vi "Get Control Terminals.vi"(8 "error in (no error)":errorcluster, 11 "VI in":refnum<vi>) -> (0 "error out":errorcluster, 2 "Controls":map{string, refnum<vi>}(c390), 3 "VI out":refnum<vi>)   [LabVIEW 2020, in "Pure Mock Class Generator.lvclass"]
uses:
  Pure Mock Class Generator.lvclass
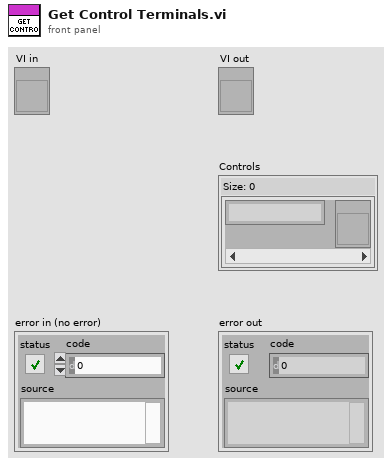
[diagram p1: front panel]
types:
  T1 = enum16{"Invalid Wire Rule", "Required", "Recommended", "Optional", "Dynamic Dispatch"}[]
  T2 = enum16{"Invalid Wire Rule", "Required", "Recommended", "Optional", "Dynamic Dispatch"}
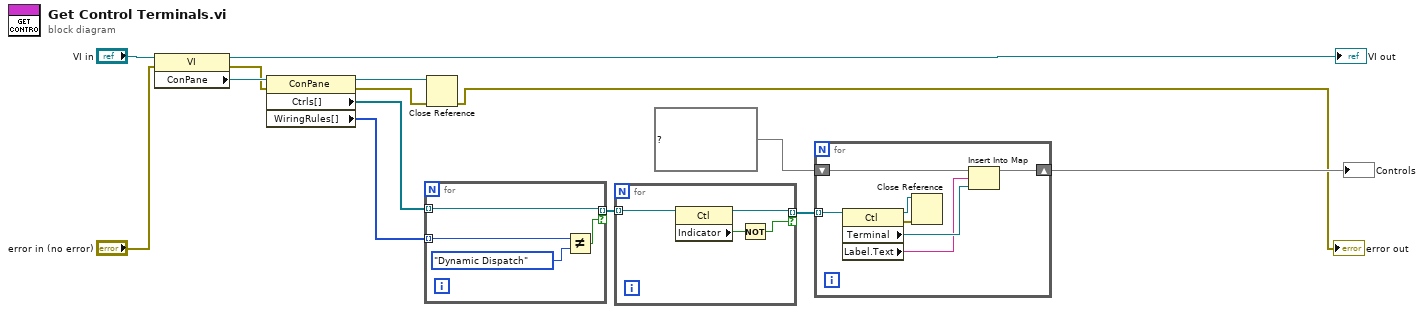
[diagram p0: block diagram]
diagram:
  n1 = property class="VI"(reference="VI in", error in="error in (no error)") -> (reference out=→"VI out":refnum<vi>, error out=w9:errorcluster, "ConPane"=w12:refnum<vi>)
  n2 = property class="ConPane"(reference=w12, error in=w9) -> (reference out=w10:refnum<vi>, error out=w11:errorcluster, "Ctrls[]"=w5:refnum<vi>[], "WiringRules[]"=w4:T1)
  n3 = for {
    tunnel: w5 -> [w16] mode=indexing
    tunnel: w4 -> [w18] mode=indexing
    tunnel: [w16] -> w3 mode=indexing if=w15
    n4 = Not Equal?(x=w18, y=T2."Dynamic Dispatch") -> (x != y?=w15:bool)
  }
  n5 = Close Reference(reference=w10, error in (no error)=w11) -> (error out=→"error out":errorcluster)
  n6 = for {
    tunnel: w3 -> [w22] mode=indexing
    tunnel: [w21] -> w2 mode=indexing if=w19
    n7 = property class="Ctl"(reference=w22) -> (reference out=w21:refnum<vi>, "Indicator"=w20:bool)  [unwired: 1 in, 1 out]
    n8 = Not(x=w20) -> (.not. x?=w19:bool)
  }
  n9 = for {
    shift-right: [w28] -> w6
    shift-left: map{string, refnum<vi>} {} ("map in") -> [w29]
    tunnel: w2 -> [w27] mode=indexing
    n10 = property class="Ctl"(reference=w27) -> (reference out=w24:refnum<vi>, error out=w25:errorcluster, "Terminal"=w26:refnum<vi>, "Label.Text"=w23:string)  [unwired: 1 in]
    n11 = Close Reference(reference=w24, error in (no error)=w25) -> ()  [unwired: 1 out]
    n12 = Insert Into Map(map in=w29, key=w23, value=w26) -> (map out=w28:map{string, refnum<vi>})  [unwired: 2 out]
  }
  "Controls" <- w6
